vi "Teleop.vi"(10 "Match Info":T1={"Autonomous Elapsed Seconds"=0.0, "TeleOp Elapsed Seconds"=0.0, "Disabled Elapsed Seconds"=0.0, "Visited Autonomous"=FALSE, "Visited TeleOp"=FALSE, "Visited Disabled"=FALSE, "Autonomous Settings"={"Autonomous Style"=enum."Independent", "VI Refnum"=refnum}}, 11 "Call Context":T2) -> ()   [LabVIEW 2015]
doc: "This VI is called for each TeleOp packet received from the DS where the robot is not disabled. It is often used to read from the joysticks and update I/O or to update setpoints for timed control loops. It should complete and return within 20 milliseconds or it may miss DS packets."
uses:
  <vilib>/Rock Robotics/WPI/DriverStation/WPI_DriverStationDerivedRobotMode.ctl
  <vilib>/Rock Robotics/WPI/DriverStation/WPI_DriverStationMatch Info.ctl
  <vilib>/Rock Robotics/Network Tables/NT Read Boolean.vi
  <vilib>/Rock Robotics/Network Tables/NT Read Number.vi
  <vilib>/Rock Robotics/WPI/Utilities/WPI_GetSetVariantRefNum.vi
  <vilib>/Rock Robotics/Network Tables/NT Write Boolean Array.vi
  <vilib>/Rock Robotics/Network Tables/NT Write Numeric Array.vi
  Robot Global Data.vi
panel:
  in  "Axes":dbl[](array[numeric])
  in  "Turn 1 for 5 seconds":bool
  in  "Drive straight -0.5 for 5 seconds":bool
  out "Sample Slider 0":dbl(slide) scale=0.0..5.0
  out "Sample Boolean 1":bool
  out "Sample Boolean 0":bool
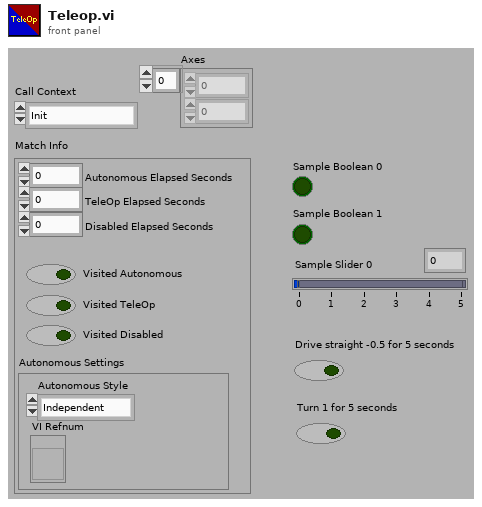
[diagram p1: front panel]
types:
  T1 = typedef "WPI_DriverStationMatch Info.ctl" = cluster{"Autonomous Elapsed Seconds":dbl, "TeleOp Elapsed Seconds":dbl, "Disabled Elapsed Seconds":dbl, "Visited Autonomous":bool, "Visited TeleOp":bool, "Visited Disabled":bool, "Autonomous Settings":cluster{"Autonomous Style":enum16{"Iterative", "Independent"}, "VI Refnum":refnum<vi>}}
  T2 = typedef "WPI_DriverStationDerivedRobotMode.ctl" = enum16{"Init", "Execute", "Stop"}
  T3 = typedef "WPI_JoystickDevRef.ctl" = cluster{"Device":T4}
  T4 = typedef "WPI_JoystickDeviceEnum.ctl" = enum16{"USB 0", "USB 1", "USB 2", "USB 3", "USB 4", "USB 5"}
  T5 = typedef "WPI_RobotDriveDevRef.ctl" = cluster{"DevStatus":errorcluster, "Motors[]":T6[], "Square Inputs":bool, "Max Output":dbl}
  T6 = typedef "WPI_MotorControlDeviceRef.ctl" = cluster{"DeviceStatus":errorcluster, "Type":T7, "PWM":cluster{"PWM Channel":T8, "DeadBand":T9}, "CAN":cluster{"Device Number":u8, "Control Mode":T10, "Semaphore":T11, "Max Vout":dbl, "TalonSRX Control Mode":T12}, "Invert":bool}
  T7 = typedef "WPI_MotorControlType.ctl" = enum16{"PWM", "CAN", "CANTalonSRX"}
  T8 = typedef "FPGA_DIOPWMChannel.ctl" = enum8{"PWM 0", "PWM 1", "PWM 2", "PWM 3", "PWM 4", "PWM 5", "PWM 6", "PWM 7", "PWM 8", "PWM 9", "PWM MXP 0", "PWM MXP 1", "PWM MXP 2", "PWM MXP 3", "PWM MXP 4", "PWM MXP 5", "PWM MXP 6", "PWM MXP 7", "PWM MXP 8", "PWM MXP 9", "Invalid"}
  T9 = typedef "WPI_PWMDeadband.ctl" = cluster{"Name":string, "maxPositivePwm":i32, "minPositivePwm":i32, "centerPwm":i32, "maxNegativePwm":i32, "minNegativePwm":i32, "angularRange":u16}
  T10 = typedef "WPI_CANJaguar_ControlMode.ctl" = enum8{"Percent VBus", "Current", "Speed", "Position", "Voltage"}
  T11 = typedef "Semaphore RefNum" = refnum<k1>
  T12 = typedef "WPI_CANTalonSRX_APIControlMode.ctl" = enum8{"Percent VBus", "Speed", "Position", "Slave", "Unchanged / Invalid", "Voltage Compensation", "Current", "Motion Profile"}
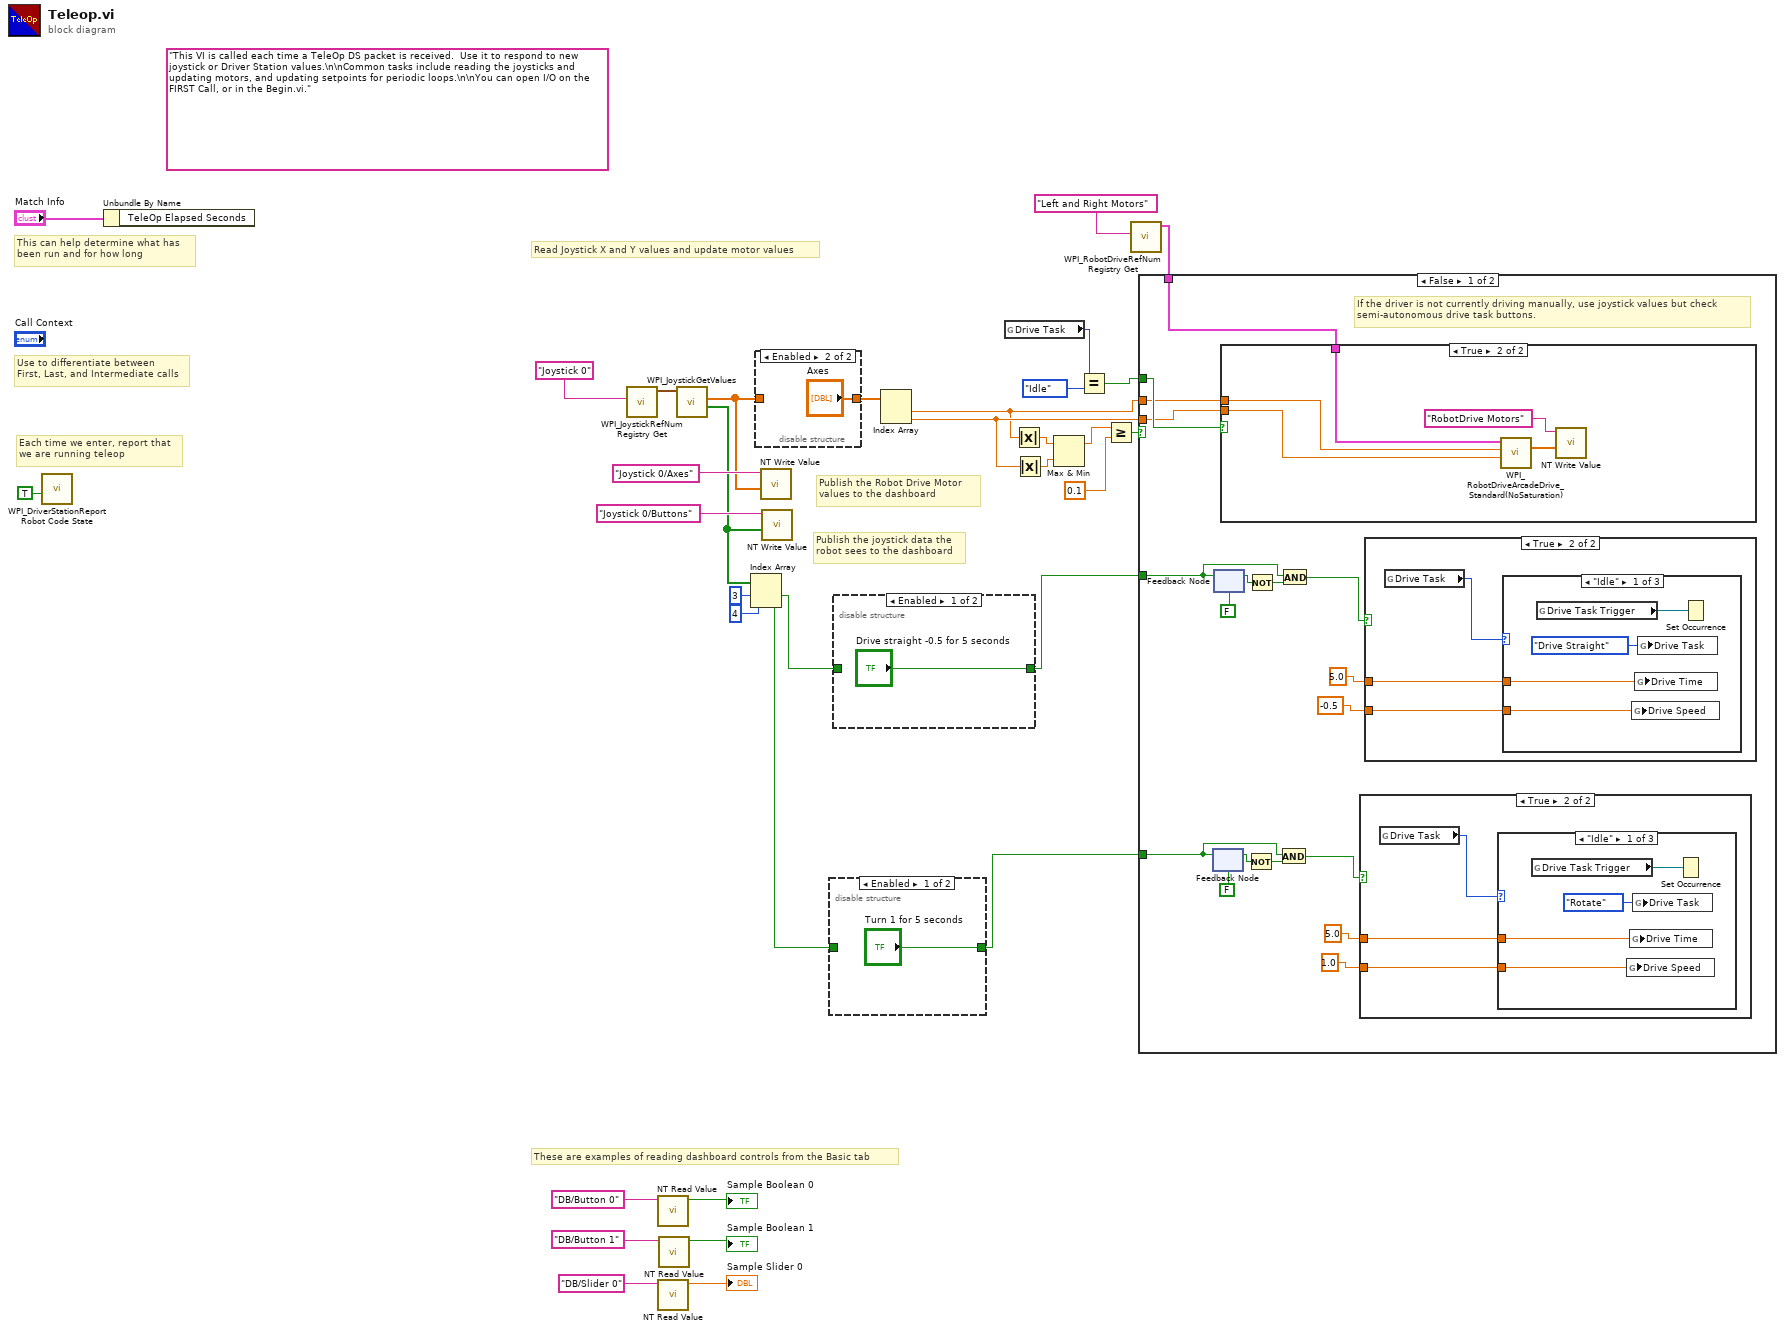
[diagram p0: block diagram]
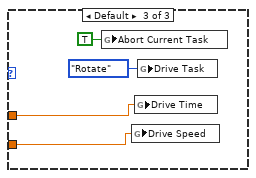
[diagram p6: hidden frame]
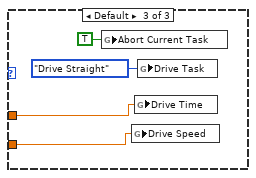
[diagram p9: hidden frame]
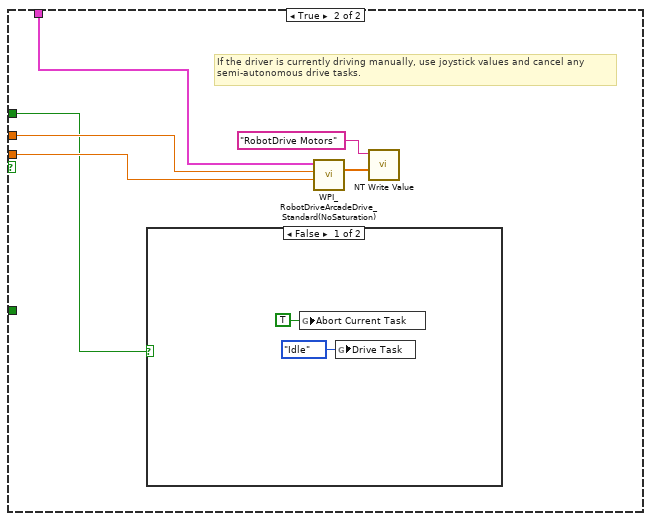
[diagram p10: hidden frame]
diagram:
  (unwired) "This VI is called each time a TeleOp DS packet is received.  Use it to respond to new joystick or Driver Station values.\n\nCommon tasks include reading the joysticks and updating motors, and updating setpoints for periodic loops.\n\nYou can open I/O on the FIRST Call, or in the Begin.vi."
  # "Publish the Robot Drive Motor\nvalues to the dashboard"
  # "Publish the joystick data the\nrobot sees to the dashboard"
  # "These are examples of reading dashboard controls from the Basic tab"
  # "Each time we enter, report that\nwe are running teleop"
  # "Use to differentiate between\nFirst, Last, and Intermediate calls"
  # "This can help determine what has\nbeen run and for how long"
  # "Read Joystick X and Y values and update motor values"
  n1 = call <vilib>:"WPI_DriverStationReport Robot Code State.vi"("TeleOp"=TRUE ("Autonomous")) -> ()  [unwired: 10 in, 1 out]
  n2 = Unbundle By Name("Match Info") -> ()  [unwired: 1 out]
  n3 = call <vilib>:"WPI_JoystickRefNum Registry Get.vi"("refnum name"="Joystick 0") -> ("JoystickDevRef"=w22:T3)  [unwired: 1 in, 9 out]
  n4 = call-poly <vilib>:"NT Read Value.vi"("Name"="DB/Button 0" ("refnum name")) -> ("Boolean"=→"Sample Boolean 0":bool)  [unwired: 9 in, 1 out]
  n5 = call-poly <vilib>:"NT Read Value.vi"("Name"="DB/Slider 0" ("refnum name")) -> ("Numeric"=→"Sample Slider 0":dbl)  [unwired: 9 in, 1 out]
  n6 = call-poly <vilib>:"NT Read Value.vi"("Name"="DB/Button 1" ("refnum name")) -> ("Boolean"=→"Sample Boolean 1":bool)  [unwired: 9 in, 1 out]
  n7 = call <vilib>:"WPI_JoystickGetValues.vi"("JoystickDevRef"=w22) -> ("Buttons"=w18:bool[], "Axes"=w4:dbl[])  [unwired: 6 in, 3 out]
  n8 = Index Array(array=w18, index #1=3 ("index"), index #2=4 ("index")) -> (element #1=w15:bool, element #2=w14:bool)
  n9 = disable-structure shown="Enabled" {
    disable-tunnel: w4 -> [w34 _]
    disable-tunnel: [w34 "Axes"] -> w3
    frame Disabled {
    }
    frame Enabled {
    }
  }
  n10 = call-poly <vilib>:"NT Write Value.vi"("Numeric Array"=w4, "Name"="Joystick 0/Axes") -> ()  [unwired: 9 in, 1 out]
  n11 = call-poly <vilib>:"NT Write Value.vi"("Boolean Array"=w18, "Name"="Joystick 0/Buttons") -> ()  [unwired: 9 in, 1 out]
  n12 = disable-structure shown="Enabled" {
    disable-tunnel: ["Turn 1 for 5 seconds" w37] -> w7
    disable-tunnel: w14 -> [_ w37]
    frame Enabled {
    }
    frame Disabled {
    }
  }
  n13 = disable-structure shown="Enabled" {
    disable-tunnel: ["Drive straight -0.5 for 5 seconds" w39] -> w8
    disable-tunnel: w15 -> [_ w39]
    frame Enabled {
    }
    frame Disabled {
    }
  }
  n14 = Index Array(array=w3) -> (element #1=w5:dbl, element #2=w6:dbl)  [unwired: 2 in]
  n15 = global read "Robot Global Data.vi" "Drive Task"() -> (w25:enum16{"Idle", "Drive Straight", "Rotate"})
  n16 = Absolute Value(x=w5) -> (abs(x)=w10:dbl)
  n17 = Absolute Value(x=w6) -> (abs(x)=w11:dbl)
  n18 = Max & Min(x=w10, y=w11) -> (max(x,y)=w12:dbl)  [unwired: 1 out]
  n19 = Equal?(x=w25, y=enum16{"Idle", "Drive Straight", "Rotate"}."Idle") -> (x = y?=w19:bool)
  n20 = Greater Or Equal?(x=w12, y=0.1) -> (x >= y?=w9:bool)
  n21 = call <vilib>:"WPI_RobotDriveRefNum Registry Get.vi"("refnum name"="Left and Right Motors") -> ("RobotDriveDevRef"=w1:T5)  [unwired: 1 in, 9 out]
  n22 = case shown="False" w9 {
    tunnel: w8 -> [w45 _]
    tunnel: w7 -> [w44 _]
    tunnel: w6 -> [w41 w88]
    tunnel: w5 -> [w42 w87]
    tunnel: w19 -> [w43 w86]
    tunnel: w1 -> [w40 w85]
    frame False {
      # "If the driver is not currently driving manually, use joystick values but check\nsemi-autonomous drive task buttons."
      n23 = feedback #1(FALSE ("0.5 for 5 seconds")) -> (w56:bool)
      n24 = feedback-in #1(w44) -> ()
      n25 = feedback #2(FALSE ("0.5 for 5 seconds")) -> (w48:bool)
      n26 = feedback-in #2(w45) -> ()
      n27 = case shown="True" w43 {
        tunnel: w42 -> [_ w60]
        tunnel: w41 -> [_ w59]
        tunnel: w40 -> [_ w58]
        frame False {
        }
        frame True {
          n28 = call <vilib>:"WPI_RobotDriveArcadeDrive_Standard(NoSaturation).vi"("Y axis value"=w59, "X axis value"=w60, "RobotDriveDevRef"=w58) -> ("Motor Values"=w62:dbl[])  [unwired: 1 in, 7 out]
          n29 = call-poly <vilib>:"NT Write Value.vi"("Numeric Array"=w62, "Name"="RobotDrive Motors") -> ()  [unwired: 9 in, 1 out]
        }
      }
      n30 = Not(x=w56) -> (.not. x?=w55:bool)
      n31 = Not(x=w48) -> (.not. x?=w47:bool)
      n32 = And(x=w44, y=w55) -> (x .and. y?=w57:bool)
      n33 = And(x=w45, y=w47) -> (x .and. y?=w49:bool)
      n34 = case shown="True" w57 {
        tunnel: 5.0 ("Drive Time") -> [_ w64]
        tunnel: 1.0 ("Drive Speed") -> [_ w63]
        frame False {
        }
        frame True {
          n35 = global read "Robot Global Data.vi" "Drive Task"() -> (w65:enum16{"Idle", "Drive Straight", "Rotate"})
          n36 = case shown="\"Idle\"" w65 {
            tunnel: w64 -> [w68 _ w73]
            tunnel: w63 -> [w67 _ w72]
            frame "Idle" {
              n37 = global read "Robot Global Data.vi" "Drive Task Trigger"() -> (w69:refnum<k4>)
              n38 = global write "Robot Global Data.vi" "Drive Speed"(w67) -> ()
              n39 = global write "Robot Global Data.vi" "Drive Time"(w68) -> ()
              n40 = global write "Robot Global Data.vi" "Drive Task"(enum16{"Idle", "Drive Straight", "Rotate"}."Rotate" ("Drive Task")) -> ()
              n41 = Set Occurrence(w69) -> ()
            }
            frame "Rotate" {
            }
            frame Default {
              n42 = global write "Robot Global Data.vi" "Abort Current Task"(TRUE ("Abort Current Task")) -> ()
              n43 = global write "Robot Global Data.vi" "Drive Speed"(w72) -> ()
              n44 = global write "Robot Global Data.vi" "Drive Time"(w73) -> ()
              n45 = global write "Robot Global Data.vi" "Drive Task"(enum16{"Idle", "Drive Straight", "Rotate"}."Rotate" ("Drive Task")) -> ()
            }
          }
        }
      }
      n46 = case shown="True" w49 {
        tunnel: 5.0 ("Drive Time") -> [_ w75]
        tunnel: -0.5 ("Drive Speed") -> [_ w74]
        frame False {
        }
        frame True {
          n47 = global read "Robot Global Data.vi" "Drive Task"() -> (w76:enum16{"Idle", "Drive Straight", "Rotate"})
          n48 = case shown="\"Idle\"" w76 {
            tunnel: w75 -> [w79 _ w84]
            tunnel: w74 -> [w78 _ w83]
            frame "Idle" {
              n49 = global read "Robot Global Data.vi" "Drive Task Trigger"() -> (w80:refnum<k4>)
              n50 = global write "Robot Global Data.vi" "Drive Speed"(w78) -> ()
              n51 = global write "Robot Global Data.vi" "Drive Time"(w79) -> ()
              n52 = global write "Robot Global Data.vi" "Drive Task"(enum16{"Idle", "Drive Straight", "Rotate"}."Drive Straight" ("Drive Task")) -> ()
              n53 = Set Occurrence(w80) -> ()
            }
            frame "Drive Straight" {
            }
            frame Default {
              n54 = global write "Robot Global Data.vi" "Abort Current Task"(TRUE ("Abort Current Task")) -> ()
              n55 = global write "Robot Global Data.vi" "Drive Speed"(w83) -> ()
              n56 = global write "Robot Global Data.vi" "Drive Time"(w84) -> ()
              n57 = global write "Robot Global Data.vi" "Drive Task"(enum16{"Idle", "Drive Straight", "Rotate"}."Drive Straight" ("Drive Task")) -> ()
            }
          }
        }
      }
    }
    frame True {
      # "If the driver is currently driving manually, use joystick values and cancel any\nsemi-autonomous drive tasks."
      n58 = case shown="False" w86 {
        frame False {
          n59 = global write "Robot Global Data.vi" "Abort Current Task"(TRUE ("Abort Current Task")) -> ()
          n60 = global write "Robot Global Data.vi" "Drive Task"(enum16{"Idle", "Drive Straight", "Rotate"}."Idle" ("Drive Task")) -> ()
        }
        frame True {
        }
      }
      n61 = call <vilib>:"WPI_RobotDriveArcadeDrive_Standard(NoSaturation).vi"("Y axis value"=w88, "X axis value"=w87, "RobotDriveDevRef"=w85) -> ("Motor Values"=w90:dbl[])  [unwired: 1 in, 7 out]
      n62 = call-poly <vilib>:"NT Write Value.vi"("Numeric Array"=w90, "Name"="RobotDrive Motors") -> ()  [unwired: 9 in, 1 out]
    }
  }
